vi "Random Number In Range.vi"(1 "Limite inférieure":u32, 2 "Limite supérieure":u32=1) -> (0 "Nb aléatoire":u32)   [LabVIEW 2009]
doc: "Renvoie un nombre aléatoire dans la gamme spécifiée par les limites supérieure et inférieure."
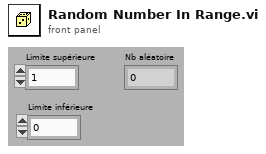
[diagram p1: front panel]
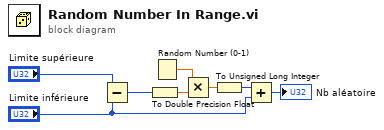
[diagram p0: block diagram]
diagram:
  n1 = Subtract ("Soustraire")(x="Limite supérieure", y="Limite inférieure") -> (x-y=w6:u32)
  n2 = To Double Precision Float ("En flottant double précision")(number=w6) -> (double precision float=w2:dbl)
  n3 = Random Number (0-1) ("Nombre aléatoire (0-1)")() -> (number: 0 to 1=w3:dbl)
  n4 = Multiply ("Multiplier")(x=w3, y=w2) -> (x*y=w8:dbl)
  n5 = To Unsigned Long Integer ("En entier long non signé")(number=w8) -> (unsigned 32bit integer=w1:u32)
  n6 = Add ("Additionner")(x=w1, y="Limite inférieure") -> (x+y=→"Nb aléatoire":u32)
